vi "indexNaPrzekatnej.vi"() -> ()   [LabVIEW 2024]
panel:
  out "out":dbl[][](array[numeric])
  in  "in":dbl[](array[numeric])
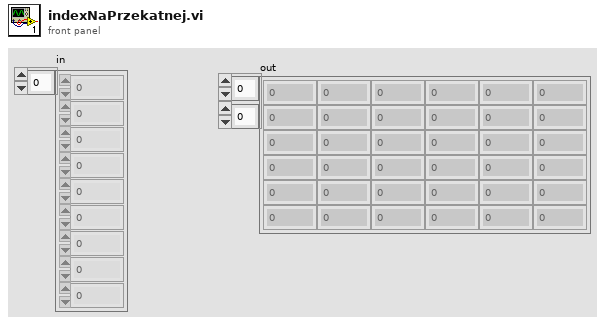
[diagram p1: front panel]
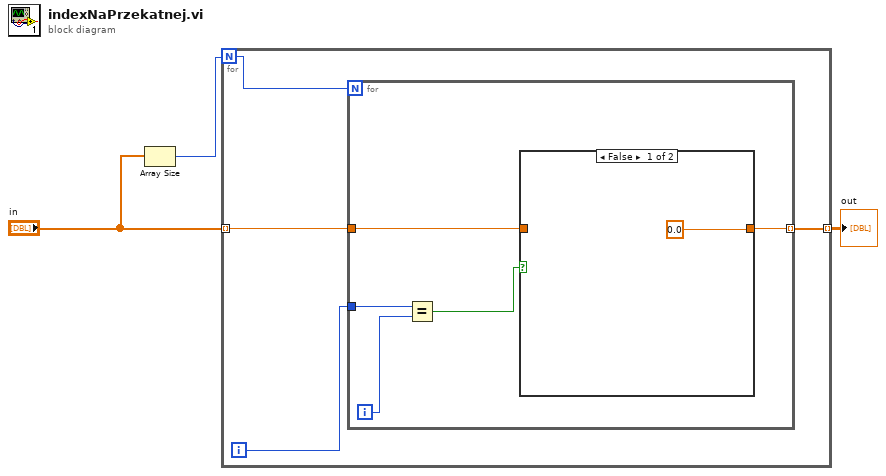
[diagram p0: block diagram]
diagram:
  n1 = Array Size(array="in") -> (size(s)=w1:i32)
  n2 = for {
    N: w1 -> [w4]
    tunnel: "in" -> [w6] mode=indexing
    tunnel: [w5] -> w3 mode=indexing
    i -> [w7]
    n3 = for {
      N: w4 -> [_]
      tunnel: w7 -> [w11]
      tunnel: w6 -> [w9]
      tunnel: [w8] -> w5 mode=indexing
      i -> [w12]
      n4 = Equal?(x=w11, y=w12) -> (x = y?=w10:bool)
      n5 = case shown="False" w10 {
        tunnel: w9 -> [_ w14]
        tunnel: [0.0 w14] -> w8
        frame False {
        }
        frame True {
        }
      }
    }
  }
  "out" <- w3
